vi "myRIO_BRig_Host_parse_dataTrial__read__getMaxTrial.vi"(0 "input_idxUnknown":i32, 1 "input_arrayUnknown":i32[][](array[numeric]), 2 "input_idxReward":i32, 3 "input_arrayReward":i32[][](array[numeric]), 4 "input_idxWrong":i32, 5 "input_arrayWrong":i32[][](array[numeric]), 6 "input_idxTimeout":i32, 7 "input_arrayTimeout":i32[][](array[numeric])) -> (21 "output_maxTrial":i32)   [LabVIEW 2014]
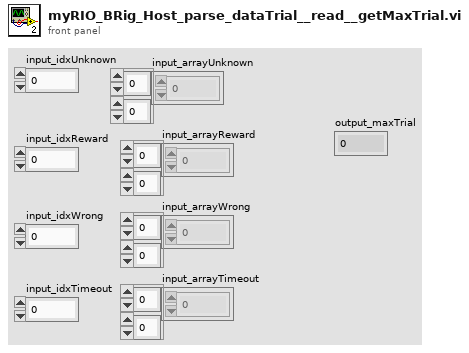
[diagram p1: front panel]
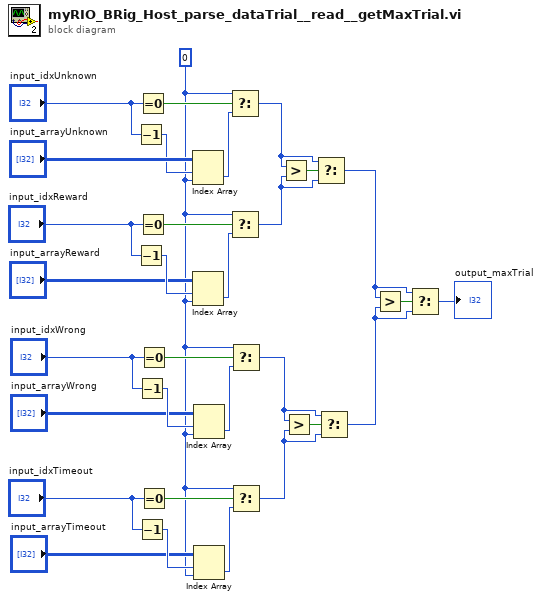
[diagram p0: block diagram]
diagram:
  w11 = 0 ("disabled index (col)")
  n1 = Decrement(x="input_idxUnknown") -> (x-1=w28:i32)
  n2 = Decrement(x="input_idxReward") -> (x-1=w25:i32)
  n3 = Decrement(x="input_idxWrong") -> (x-1=w20:i32)
  n4 = Decrement(x="input_idxTimeout") -> (x-1=w15:i32)
  n5 = Equal To 0?(x="input_idxUnknown") -> (x = 0?=w31:bool)
  n6 = Equal To 0?(x="input_idxReward") -> (x = 0?=w26:bool)
  n7 = Equal To 0?(x="input_idxWrong") -> (x = 0?=w21:bool)
  n8 = Equal To 0?(x="input_idxTimeout") -> (x = 0?=w16:bool)
  n9 = Index Array(array="input_arrayUnknown", index (row)=w28, index (col)=w11) -> (element=w27:i32)
  n10 = Index Array(array="input_arrayReward", index (row)=w25, index (col)=w11) -> (element=w24:i32)
  n11 = Index Array(array="input_arrayWrong", index (row)=w20, index (col)=w11) -> (element=w19:i32)
  n12 = Index Array(array="input_arrayTimeout", index (row)=w15, index (col)=w11) -> (element=w14:i32)
  n13 = Select(t=w11, s=w31, f=w27) -> (s? t:f=w9:i32)
  n14 = Select(t=w11, s=w26, f=w24) -> (s? t:f=w8:i32)
  n15 = Select(t=w11, s=w21, f=w19) -> (s? t:f=w5:i32)
  n16 = Select(t=w11, s=w16, f=w14) -> (s? t:f=w6:i32)
  n17 = Greater?(x=w9, y=w8) -> (0:w10:bool)
  n18 = Greater?(x=w5, y=w6) -> (0:w7:bool)
  n19 = Select(t=w9, s=w10, f=w8) -> (s? t:f=w3:i32)
  n20 = Select(t=w5, s=w7, f=w6) -> (s? t:f=w2:i32)
  n21 = Greater?(x=w3, y=w2) -> (0:w4:bool)
  n22 = Select(t=w3, s=w4, f=w2) -> (s? t:f=→"output_maxTrial":i32)
